vi "Losu pozycje.vi"(8 "error in (no error)":errorcluster, 11 "Swiat in":refnum<class "Swiat.lvclass">) -> (0 "error out":errorcluster, 2 "Random Position":T1, 3 "Swiat out":refnum<class "Swiat.lvclass">)   [LabVIEW 2014, in "Swiat.lvclass"]
uses:
  Swiat.lvclass
  Typedefs/Position.ctl
  Swiat.lvclass/Swiat.ctl
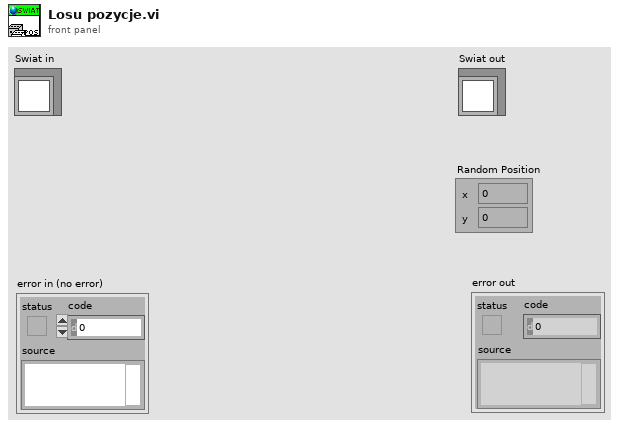
[diagram p1: front panel]
types:
  T1 = typedef "Position.ctl" = cluster{"x":i16, "y":i16}
  T2 = typedef "LVBoundsTypeDef.ctl" = cluster{"Width":u32, "Height":u32}
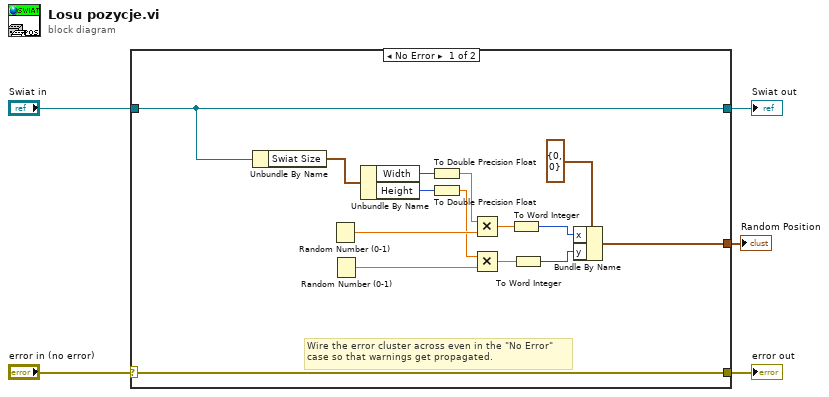
[diagram p0: block diagram]
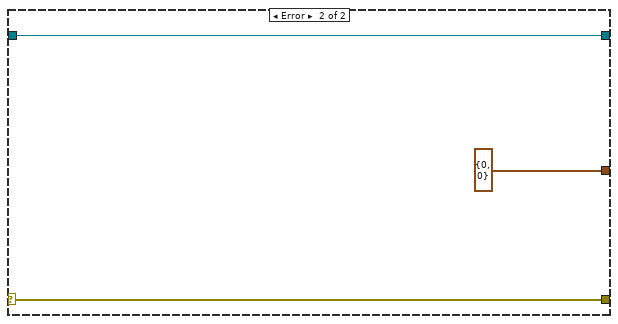
[diagram p2: hidden frame]
diagram:
  n1 = case shown="No Error" "error in (no error)" {
    selector: "error in (no error)" -> [w20 w23]
    tunnel: [w20 w23] -> w4
    tunnel: [w19 w22] -> w2
    tunnel: "Swiat in" -> [w19 w22]
    tunnel: [w6 T1 {"x"=0, "y"=0} ("Position")] -> w1
    frame No Error {
      # "Wire the error cluster across even in the \"No Error\"\ncase so that warnings get propagated."
      n2 = Unbundle By Name(w19) -> ("Swiat Size"=w18:T2)
      n3 = Random Number (0-1)() -> (number: 0 to 1=w17:dbl)
      n4 = Random Number (0-1)() -> (number: 0 to 1=w12:dbl)
      n5 = Unbundle By Name(w18) -> ("Width"=w16:u32, "Height"=w15:u32)
      n6 = To Double Precision Float(number=w16) -> (double precision float=w14:dbl)
      n7 = To Double Precision Float(number=w15) -> (double precision float=w13:dbl)
      n8 = Multiply(x=w14, y=w17) -> (x*y=w10:dbl)
      n9 = Multiply(x=w13, y=w12) -> (x*y=w9:dbl)
      n10 = To Word Integer(number=w10) -> (16bit integer=w8:i16)
      n11 = To Word Integer(number=w9) -> (16bit integer=w7:i16)
      n12 = Bundle By Name(cluster=T1 {"x"=0, "y"=0} ("Position"), "x"=w8, "y"=w7) -> (w6:T1)
    }
    frame Error {
    }
  }
  "error out" <- w4
  "Swiat out" <- w2
  "Random Position" <- w1
